vi "IED Test Launcher.vi"() -> ()   [LabVIEW 2016, in "IED Test Framework.lvlib"]
uses:
  IED Test Framework.lvlib
  IED Test/Controls/Tests Cluster.ctl
  IED Test/IED Test.lvclass
  C:/Program Files (x86)/National Instruments/LabVIEW 2016/vi.lib/ActorFramework/Actor/Actor.lvclass
  <vilib>/ActorFramework/Actor/Actor.lvclass
  <vilib>/RTI DDS Toolkit/Library/LVDDS_library.lvlib
panel:
  in  "Tests":T1
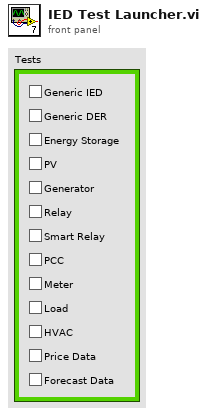
[diagram p1: front panel]
types:
  T1 = typedef "IED Test Framework.lvlib/IED Test.lvclass/Tests Cluster.ctl" = cluster{"Generic IED":bool, "Generic DER":bool, "Energy Storage":bool, "PV":bool, "Generator":bool, "Relay":bool, "Smart Relay":bool, "PCC":bool, "Meter":bool, "Load":bool, "HVAC":bool, "Price Data":bool, "Forecast Data":bool}
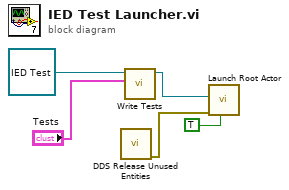
[diagram p0: block diagram]
diagram:
  n1 = call <vilib>:"DDS Release Unused Entities.vi"() -> ("error out"=w1:errorcluster)  [unwired: 10 in, 1 out]
  n2 = call-dynamic "Write Tests.vi"("Tests"="Tests", "IED Test in"=refnum<class "IED Test.lvclass"> refnum ("IED Test Framework.lvlib:IED Test.lvclass")) -> ("IED Test out"=w3:refnum<class "IED Test.lvclass">)  [unwired: 9 in]
  n3 = call <vilib>:"Launch Root Actor.vi"("Open Actor Core front panel? (F)"=TRUE, "error in (no error)"=w1, "Actor"=w3) -> ()  [unwired: 7 in, 2 out]
